vi "shift 2D image arrayin.vi"(0 "Array in":dbl[][](array[numeric]), 1 "shift":i32[](array[numeric])) -> (2 "Array out":dbl[][](array[numeric]))   [LabVIEW 2018]
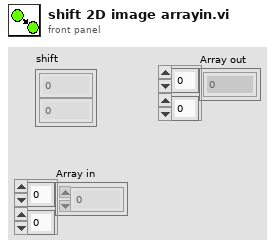
[diagram p1: front panel]
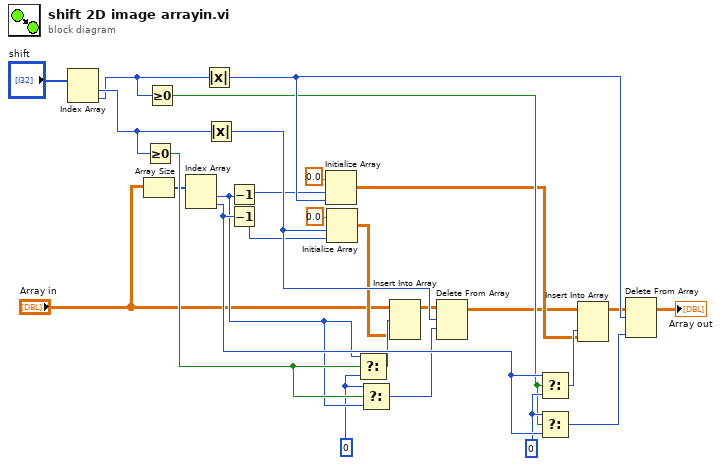
[diagram p0: block diagram]
diagram:
  w22 = 0 ("index (row)")
  w16 = 0 ("index (row)")
  n1 = Index Array(array="shift") -> (element #1=w2:i32, element #2=w1:i32)  [unwired: 2 in]
  n2 = Array Size(array="Array in") -> (size(s)=w5:i32[])
  n3 = Greater Or Equal To 0?(x=w2) -> (x >= 0?=w20:bool)
  n4 = Greater Or Equal To 0?(x=w1) -> (x >= 0?=w21:bool)
  n5 = Index Array(array=w5) -> (element #1=w17:i32, element #2=w23:i32)  [unwired: 2 in]
  n6 = Absolute Value(x=w1) -> (abs(x)=w26:i32)
  n7 = Absolute Value(x=w2) -> (abs(x)=w27:i32)
  n8 = Decrement(x=w17) -> (x-1=w14:i32)
  n9 = Decrement(x=w23) -> (x-1=w15:i32)
  n10 = Initialize Array(0.0 ("element"), w14, w26) -> (w13:dbl[][])
  n11 = Initialize Array(0.0 ("element"), w27, w15) -> (w7:dbl[][])
  n12 = Select(t=w17, s=w20, f=w16) -> (s? t:f=w19:i32)
  n13 = Select(t=w16, s=w20, f=w17) -> (s? t:f=w18:i32)
  n14 = Insert Into Array(array="Array in", index (row)=w19, new element=w7) -> (w8:dbl[][])  [unwired: 1 in]
  n15 = Delete From Array(array=w8, length=w27, index (row)=w18) -> (array with subset deleted=w10:dbl[][])  [unwired: 1 in, 1 out]
  n16 = Select(t=w23, s=w21, f=w22) -> (s? t:f=w24:i32)
  n17 = Select(t=w22, s=w21, f=w23) -> (s? t:f=w25:i32)
  n18 = Insert Into Array(array=w10, index (col)=w24, new element=w13) -> (w9:dbl[][])  [unwired: 1 in]
  n19 = Delete From Array(array=w9, length=w26, index (col)=w25) -> (array with subset deleted=→"Array out":dbl[][])  [unwired: 1 in, 1 out]
